vi "Convert Voltage to Angle-with AssertAPI Assertions.vi"(10 "Inclinometer output (V)":dbl) -> (2 "Angle":dbl)   [LabVIEW 2018]
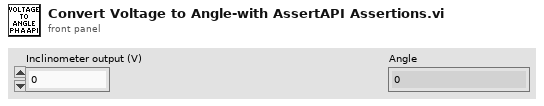
[diagram p1: front panel]
types:
  T1 = typedef "dbl.ctl" = dbl
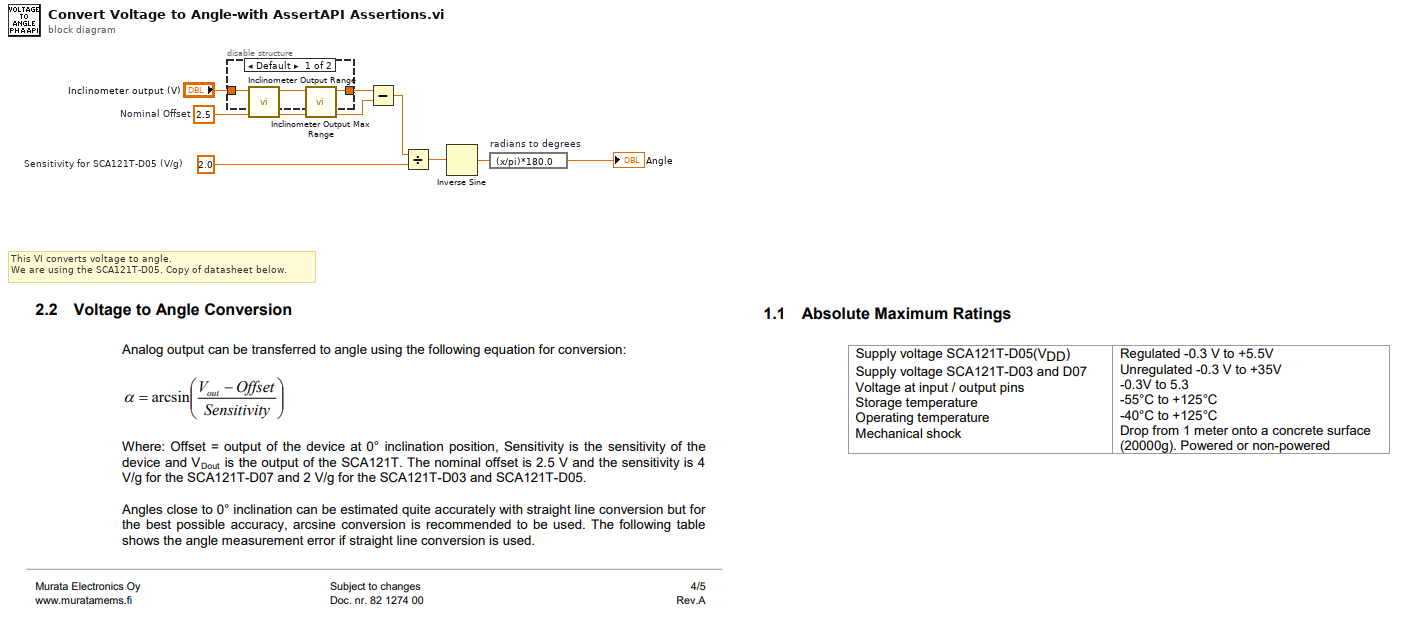
[diagram p0: block diagram]
diagram:
  w4 = 2.5  # Nominal Offset
  w7 = 2.0  # Sensitivity for SCA121T-D05 (V/g)
  # "This VI converts voltage to angle.\nWe are using the SCA121T-D05. Copy of datasheet below."
  n1 = disable-structure shown="Default" {
    disable-tunnel: "Inclinometer output (V)" -> [w11 w12]
    disable-tunnel: [w9 w12] -> w1
    frame condition #0 (active) {
      n2 = call "Inclinometer Output Range.vi"("Data In"=w11) -> ("Data Out"=w10:T1)  [unwired: 10 in]
      n3 = call "Inclinometer Output Max Range.vi"("Data In"=w10) -> ("Data Out"=w9:T1)  [unwired: 10 in]
    }
    frame condition #1 {
    }
  }
  n4 = Subtract(x=w1, y=w4) -> (x-y=w6:T1)
  n5 = Divide(x=w6, y=w7) -> (x/y=w8:T1)
  n6 = Inverse Sine(1:w8) -> (0:w3:T1)
  n7 = expression code="(x/pi)*180.0" "radians to degrees"(w3) -> (→"Angle":T1)
